vi "将相关实验数据存入tdms文件.vi"(7 "实验数据-数组":dbl[](array[numeric]), 9 "channel":string[](array[string]), 10 "group":string, 11 "file path":path) -> ()   [LabVIEW 2018]
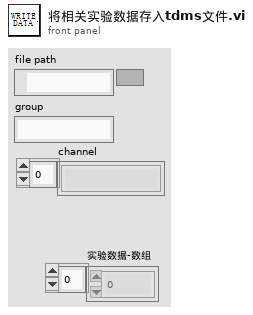
[diagram p1: front panel]
types:
  T1 = enum16{"open", "open or create", "create or replace", "create", "open (read-only)"}
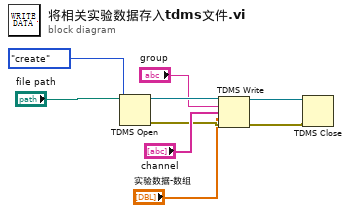
[diagram p0: block diagram]
diagram:
  n1 = TDMS Open(10:T1."create" ("operation (0:open)"), 11:"file path") -> (0:w4:errorcluster, 3:w7:refnum<k34>)  [unwired: 5 in]
  n2 = TDMS Write(0:w7, 5:"group", 7:"channel", 9:"实验数据-数组", 11:w4) -> (4:w2:refnum<k34>, 15:w1:errorcluster)  [unwired: 1 in, 2 out]
  n3 = TDMS Close(8:w1, 11:w2) -> ()  [unwired: 2 out]
